vi "_InputName to JKISM Mode.vi"(11 "String":string) -> (1 "QName":string, 2 "JKISM Mode":T1, 3 "String(dup)":string)   [LabVIEW 2014, in "JKI-State-Machine-Plus.lvlib"]
uses:
  JKI-State-Machine-Plus.lvlib
  Typedef/_JKISM_MODE.ctl
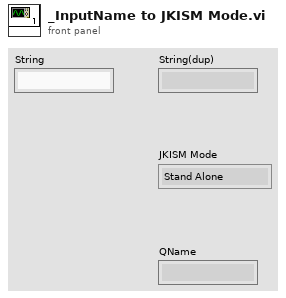
[diagram p1: front panel]
types:
  T1 = typedef "JKI-State-Machine-Plus.lvlib/_JKISM_MODE.ctl" = enum16{"Stand Alone", "JKISM", "Dispatch Worker"}
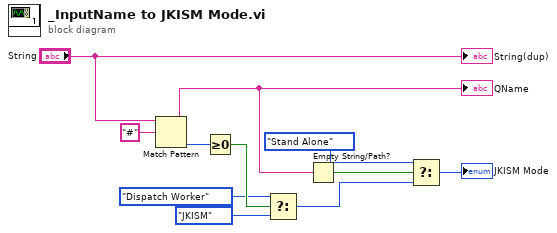
[diagram p0: block diagram]
diagram:
  n1 = Match Pattern(string="String", regular expression="#") -> (before substring=w3:string, offset past match=w9:i32)  [unwired: 1 in, 2 out]
  "QName" <- w3
  n2 = Greater Or Equal To 0?(x=w9) -> (x >= 0?=w8:bool)
  n3 = Select(t=_JKISM_MODE."Dispatch Worker" ("Mode"), s=w8, f=_JKISM_MODE."JKISM" ("Mode")) -> (s? t:f=w4:T1)
  n4 = Empty String/Path?(string/path=w3) -> (empty?=w1:bool)
  n5 = Select(t=_JKISM_MODE."Stand Alone" ("Mode"), s=w1, f=w4) -> (s? t:f=→"JKISM Mode":T1)
  "String(dup)" <- "String"
